vi "AttrGetTxPendingMsg.vi"(8 "error in":errorcluster, 11 "CanHandleIn":T1) -> (0 "error out":errorcluster, 2 "Value":u32, 3 "CanHandleOut":T1)   [LabVIEW 2011, in "Konvolucio MCAN120803.lvlib"]
uses:
  <instrlib>/Konvolucio MCAN120803/Konvolucio MCAN120803.lvlib
  <instrlib>/Konvolucio MCAN120803/Types/CanHandleType.ctl
  C:/Program Files/National Instruments/LabVIEW 2011/instr.lib/Konvolucio MCAN120803/Private/Konvolucio.MCAN120803.API.dll
  Private/Konvolucio.MCAN120803.API.dll
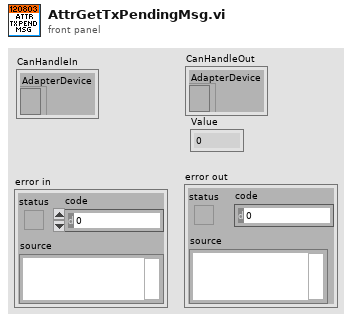
[diagram p1: front panel]
types:
  T1 = typedef "Konvolucio MCAN120803.lvlib/CanHandleType.ctl" = cluster{"AdapterDevice":refnum<k24>}
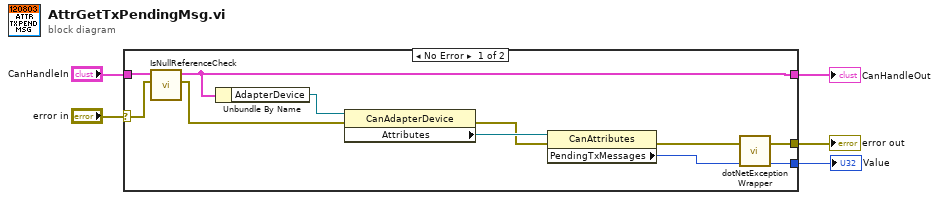
[diagram p0: block diagram]
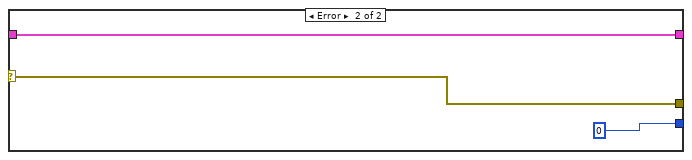
[diagram p2: hidden frame]
diagram:
  n1 = case shown="No Error" "error in" {
    selector: "error in" -> [w13 w18]
    tunnel: [w15 w18] -> w5
    tunnel: [w11 0 ("Attributes.PendingMessages")] -> w4
    tunnel: "CanHandleIn" -> [w14 w16]
    tunnel: [w12 w16] -> w2
    frame No Error {
      n2 = call <instrlib>:"IsNullReferenceCheck.vi"("error in"=w13, "MCanHandleIn"=w14) -> ("error out"=w8:errorcluster, "MCanHandleOut"=w12:T1)  [unwired: 5 in]
      n3 = Unbundle By Name(w12) -> ("AdapterDevice"=w9:refnum<k24>)
      n4 = property class="CanAdapterDevice"(reference=w9, error in=w8) -> (error out=w6:errorcluster, "Attributes"=w7:refnum<k24>)  [unwired: 1 out]
      n5 = property class="CanAttributes"(reference=w7, error in=w6) -> (error out=w10:errorcluster, "PendingTxMessages"=w11:u32)  [unwired: 1 out]
      n6 = call <instrlib>:"dotNetExceptionWrapper.vi"("error in"=w10) -> ("error out"=w15:errorcluster)  [unwired: 2 in]
    }
    frame Error {
    }
  }
  "error out" <- w5
  "Value" <- w4
  "CanHandleOut" <- w2
